vi "End.vi"(8 "error in (no error)":errorcluster, 11 "Channel in":refnum<class "Channel.lvclass">) -> (0 "error out":errorcluster, 3 "Channel out":refnum<class "Channel.lvclass">)   [LabVIEW 2018, in "Channel.lvclass"]
uses:
  Channel.lvclass
  Channel.lvclass/Channel.ctl
  Interface/Interface.lvclass
  <vilib>/Utility/config.llb/NI_LVConfig.lvlib
  <vilib>/Utility/config.llb/Write Key (String).vi
panel:
  out "file path":path
  out "JSON string":string
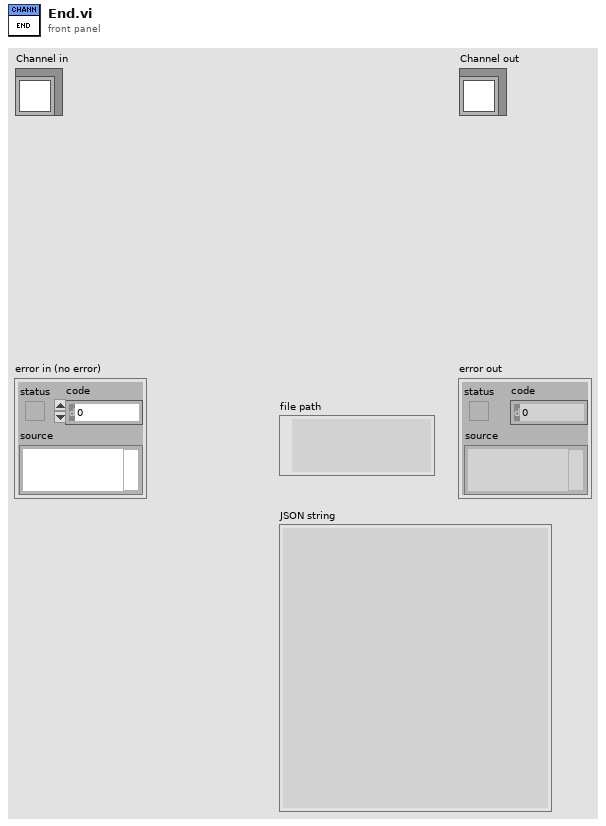
[diagram p1: front panel]
types:
  T1 = cluster{"ACQUISITION_MODE":u8, "TRIGGER_MODE":u8, "READ_MODE":u8, "PREAMP":u8, "READOUT_RATE":u8, "VERTICAL_SHIFT_SPEED":u8, "EM_MODE":u8, "EM_GAIN":u16, "SHUTTER_MODE":u8, "SHUTTER_TTL":u8, "SHUTTER_OPENING_TIME":u16, "SHUTTER_CLOSING_TIME":u16, "VBIN":u16, "HBIN":u16, "INITIAL_LINE":u16, "INITIAL_COLUMN":u16, "FINAL_LINE":u16, "FINAL_COLUMN":u16, "FRAME_TRANSFER":bool, "VERTICAL_CLOCK_VOLTAGE":u8, "AD_CHANNEL":u32}
  T2 = typedef "NI_LVConfig.lvlib/Config Data RefNum.ctl" = refnum<k1>
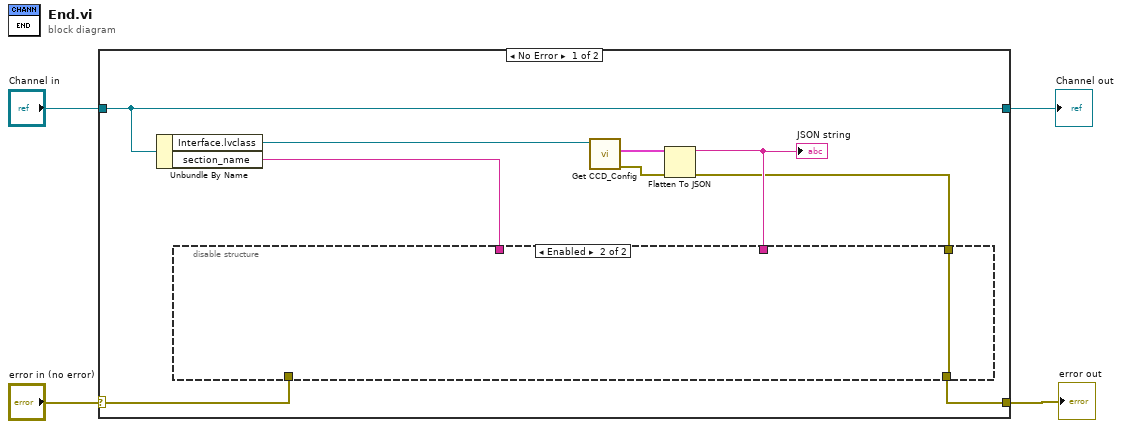
[diagram p0: block diagram]
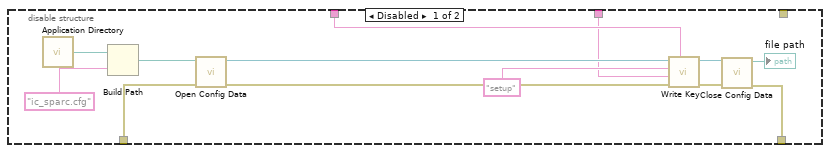
[diagram p2: hidden frame]
diagram:
  n1 = case shown="No Error" "error in (no error)" {
    selector: "error in (no error)" -> [w6 w29]
    tunnel: [w7 w29] -> w3
    tunnel: [w11 w28] -> w1
    tunnel: "Channel in" -> [w11 w28]
    frame No Error {
      n2 = Unbundle By Name(w11) -> ("Interface.lvclass"=w13:refnum<class "Interface.lvclass">, "section_name"=w9:string)
      n3 = call-dynamic "Get CCD_Config.vi"("Interface in"=w13) -> ("error out"=w10:errorcluster, "output cluster"=w12:T1)  [unwired: 8 in, 1 out]
      n4 = Flatten To JSON(anything=w12, error in (no error)=w10) -> (JSON string=w8:string, 11:w5:errorcluster)  [unwired: 1 in]
      "JSON string" <- w8
      n5 = disable-structure shown="Enabled" {
        disable-tunnel: w6 -> [w23 _]
        disable-tunnel: w9 -> [w20 _]
        disable-tunnel: w8 -> [w19 _]
        disable-tunnel: [w16 w27] -> w7
        disable-tunnel: w5 -> [_ w27]
        frame Disabled {
          n6 = call <vilib>:"Application Directory.vi"() -> ("Application Directory"=w26:path)
          n7 = Build Path(base path=w26, name or relative path="ic_sparc.cfg") -> (appended path=w24:path)
          n8 = call <vilib>:"Open Config Data.vi"("error in (no error)"=w23, "configuration file path"=w24) -> ("error out"=w14:errorcluster, "refnum"=w21:T2)  [unwired: 7 in, 1 out]
          n9 = call-poly <vilib>:"Write Key.vi"("section"=w20, "error in (no error)"=w14, "value"=w19, "key"="setup", "refnum"=w21) -> ("error out"=w17:errorcluster, "refnum out"=w18:T2)  [unwired: 4 in, 1 out]
          n10 = call <vilib>:"Close Config Data.vi"("error in (no error)"=w17, "refnum"=w18) -> ("error out"=w16:errorcluster, "file path"=→"file path":path)  [unwired: 8 in]
        }
        frame Enabled {
        }
      }
    }
    frame Error {
    }
  }
  "error out" <- w3
  "Channel out" <- w1
